vi "Write htx.vi"(8 "error in (no error)":errorcluster, 10 "htx":dbl, 11 "Update TEC Multipliers in":refnum<class "Update TEC Multipliers.lvclass">) -> (0 "error out":errorcluster, 3 "Update TEC Multipliers out":refnum<class "Update TEC Multipliers.lvclass">)   [LabVIEW 2014, in "TE Cooler.lvlib" / "Update TEC Multipliers.lvclass"]
uses:
  Update TEC Multipliers.lvclass
  Update TEC Multipliers.lvclass/Update TEC Multipliers.ctl
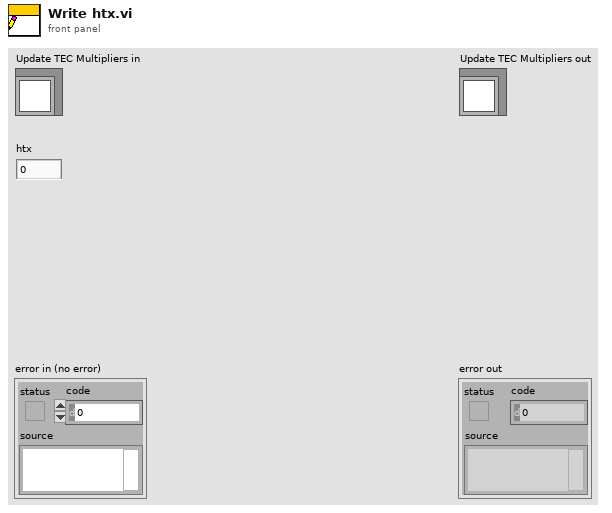
[diagram p1: front panel]
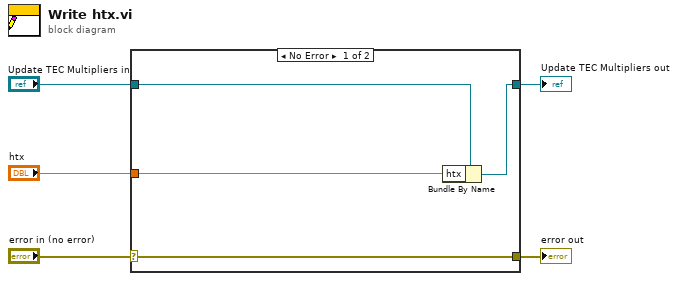
[diagram p0: block diagram]
diagram:
  n1 = case shown="No Error" "error in (no error)" {
    selector: "error in (no error)" -> [w9 w10]
    tunnel: [w9 w10] -> w4
    tunnel: [w7 w11] -> w2
    tunnel: "Update TEC Multipliers in" -> [w8 w11]
    tunnel: "htx" -> [w6 _]
    frame No Error {
      n2 = Bundle By Name(cluster=w8, "htx"=w6) -> (w7:refnum<class "Update TEC Multipliers.lvclass">)
    }
    frame Error {
    }
  }
  "error out" <- w4
  "Update TEC Multipliers out" <- w2
